vi "TEST flattening.vi"() -> ()   [LabVIEW 2011]
panel:
  in  "Numeric":i32
  out "string":string
  out "unsigned byte array":u8[](array[numeric]) format="%.0x"
  out "data string":string
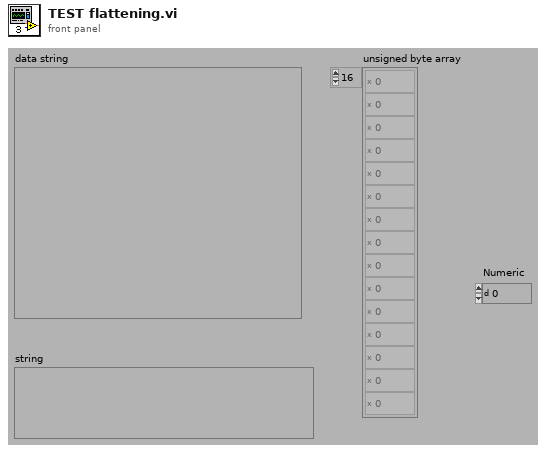
[diagram p1: front panel]
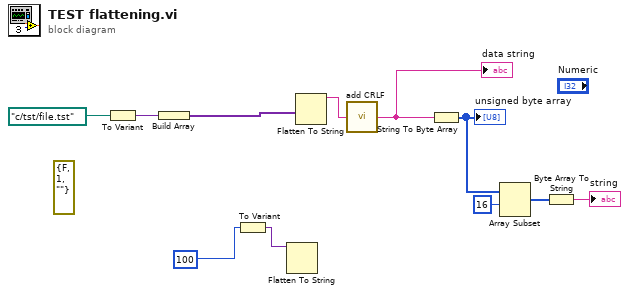
[diagram p0: block diagram]
diagram:
  (unwired) errorcluster {FALSE, 1, ""}
  n1 = To Variant(anything=path "c:/tst/file.tst") -> (Variant=w5:variant)
  n2 = Build Array(w5) -> (w2:variant[])
  n3 = To Variant(anything=100) -> (Variant=w3:variant)
  n4 = Flatten To String(anything=w3) -> ()  [unwired: 1 in, 5 out]
  n5 = Flatten To String(anything=w2) -> (data string=w7:string)  [unwired: 1 in, 4 out]
  n6 = call "add CRLF.vi"("Flattened Data"=w7) -> ("Data w/CRLF"=w1:string)  [unwired: 4 out]
  "data string" <- w1
  n7 = String To Byte Array(string=w1) -> (unsigned byte array=w11:u8[])
  "unsigned byte array" <- w11
  n8 = Array Subset(array=w11, index=16) -> (w9:u8[])  [unwired: 1 in]
  n9 = Byte Array To String(unsigned byte array=w9) -> (string=→"string":string)
